vi "Kelvinox_Rotator_Queue_Commands.vi"(1 "Control":T1 {"Angle SP" format="%#.2g"}, 3 "Queue":refnum<queue>) -> (0 "New Status":T1 {"Angle SP" format="%#.2g"})   [LabVIEW 2019]
uses:
  Kelvinox/Kelvinox_Rotator_Control.ctl
panel:
  # "Kelvinox Rotator"
  # "Kelvinox Rotator"
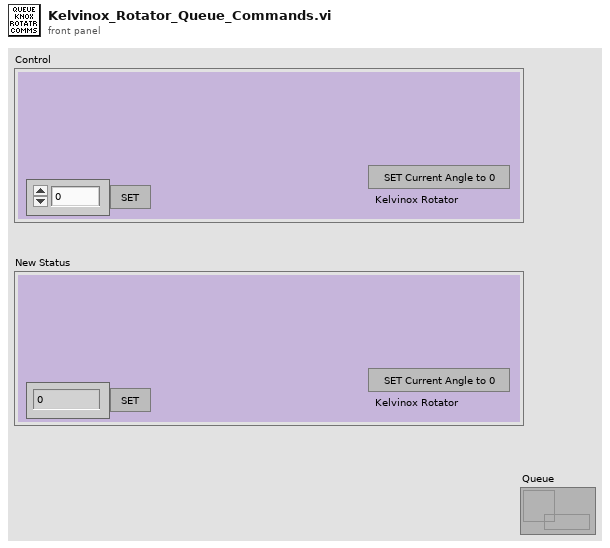
[diagram p1: front panel]
types:
  T1 = typedef "Kelvinox_Rotator_Control.ctl" = cluster{"Angle SP":dbl, "Set Angle SP":bool, "Set Angle to Zero":bool}
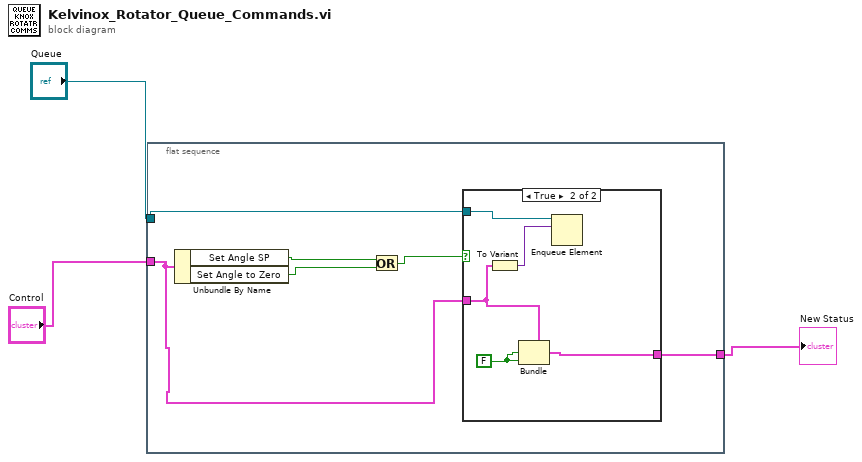
[diagram p0: block diagram]
diagram:
  n1 = flat-sequence {
    tunnel: "Queue" -> [w9]
    tunnel: "Control" -> [w5]
    tunnel: [w8] -> w1
    frame #0 {
      n2 = Unbundle By Name(w5) -> ("Set Angle SP"=w7:bool, "Set Angle to Zero"=w4:bool)
      n3 = Or(x=w7, y=w4) -> (x .or. y?=w6:bool)
      n4 = case shown="True" w6 {
        tunnel: w9 -> [_ w15]
        tunnel: w5 -> [w10 w13]
        tunnel: [w10 w12] -> w8
        frame False {
        }
        frame True {
          w11 = FALSE
          n5 = To Variant(anything=w13) -> (Variant=w14:variant)
          n6 = Bundle(cluster=w13, "Set Angle SP"=w11, "Set Angle to Zero"=w11) -> (w12:T1)  [unwired: 1 in]
          n7 = Enqueue Element(queue=w15, element=w14) -> ()  [unwired: 2 in, 3 out]
        }
      }
    }
  }
  "New Status" <- w1
